vi "term_project.vi"() -> ()   [LabVIEW 2019]
uses:
  <vilib>/userdefined/High Color/IMAQdx.ctl
  <vilib>/Utility/file.llb/Read Delimited Spreadsheet (DBL).vi
  <vilib>/vision/driver/NI_Vision_Acquisition_Software.lvlib
  <vilib>/vision/NI_Vision_Development_Module.lvlib
panel:
  in  "Choose an Action":u16(ring) items=["RGB to Gray Conversion", "Gray to RGB Conversion", "Video Processing"]
  in  "Term Project Group 2":T1(tab)
  out "Time Passed (ms)":u32
  in  "Image Path RGBG":path=path "resources/lenacolored.png"
  out "Processed Gray Scale Image":T2(plugin-control)
  out "RGB Image":T2(plugin-control)
  out "Time Passed Labview (ms)":u32
  out "Labview Gray Scale Image":T2(plugin-control)
  in  "Colormap Circular Shift":i16(slide) scale=0.0..255.0
  out "Gray Scale Image":T2(plugin-control)
  out "Colored Image":T2(plugin-control)
  in  "Colormap File Path GRGB":path=path "resources/jet.csv"
  in  "Image Path GRGB":path=path "resources/lena.png"
  out "Time Passed":u32
  in  "Colormap Shift":i16(slide) scale=0.0..255.0
  in  "stop":bool
  in  "Choose Camera":T3="cam0"
  in  "Colormap File Path For Video":path=path "resources/parula.csv"
  out "Reproduced Image with Colormap":T2(plugin-control)
  out "Processed Image":T2(plugin-control)
  out "Captured Image":T2(plugin-control)
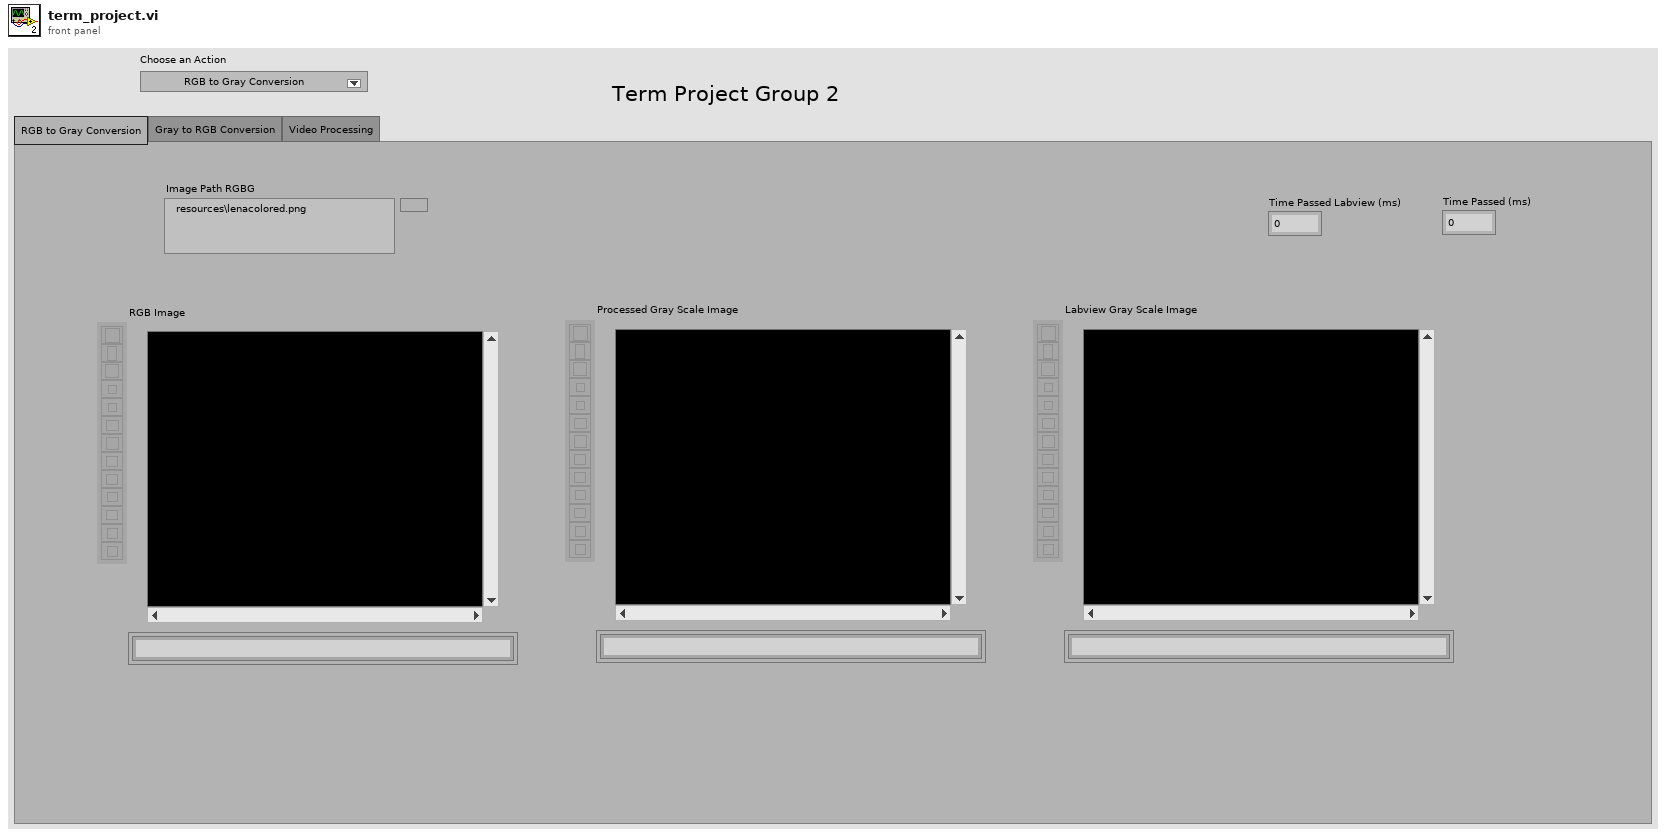
[diagram p1: front panel]
types:
  T1 = enum32{"RGB to Gray Conversion", "Gray to RGB Conversion", "Video Processing"}
  T2 = typedef "IMAQ Image.ctl" = refnum<image>
  T3 = typedef "IMAQdx.ctl" = refnum<k21>
  T4 = typedef "Image Type" = u32
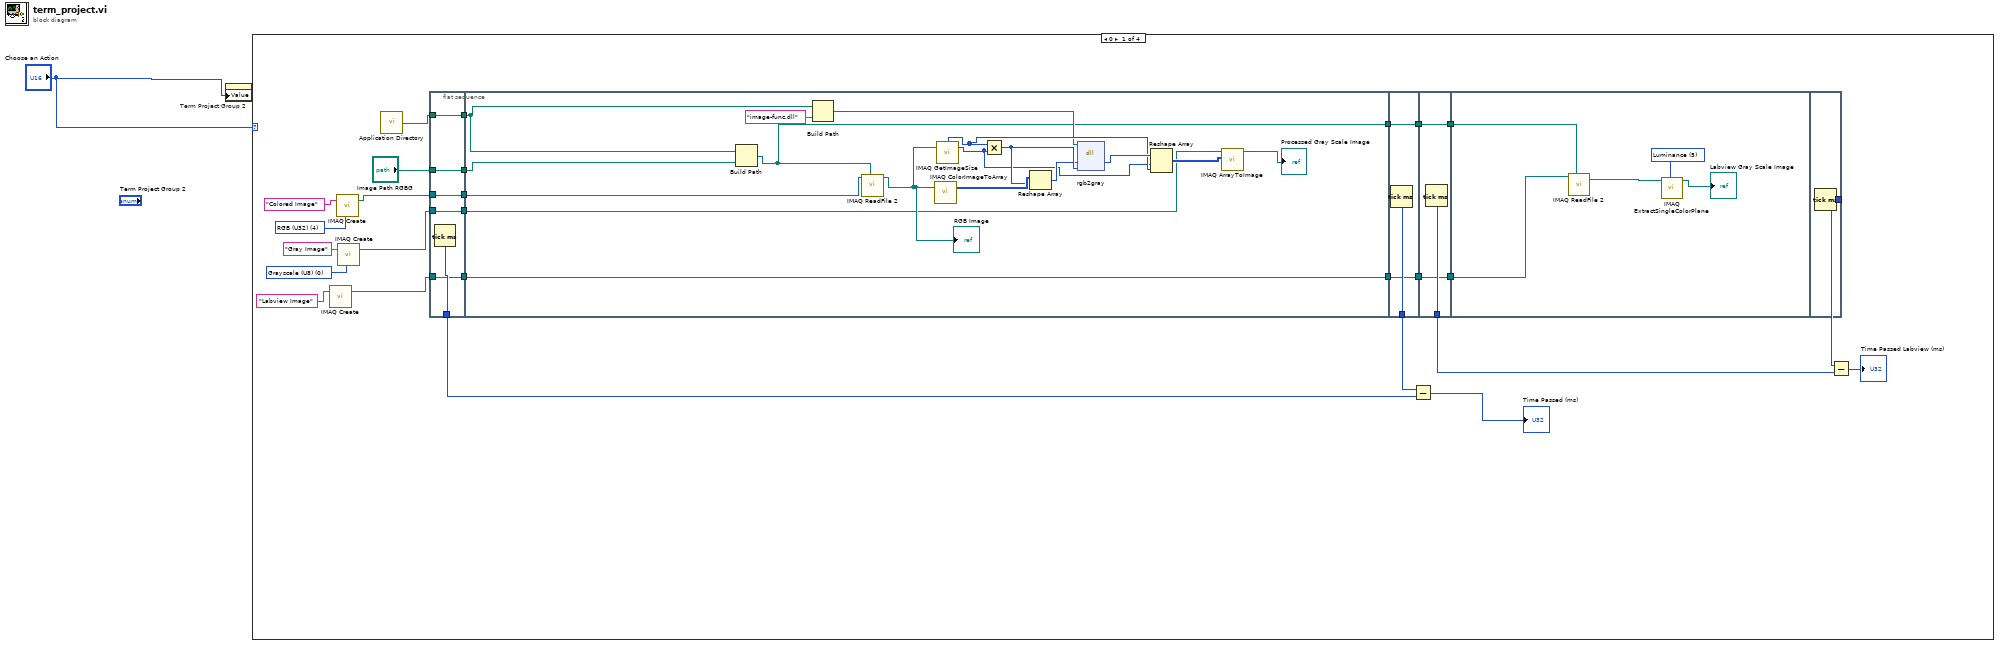
[diagram p0: block diagram]
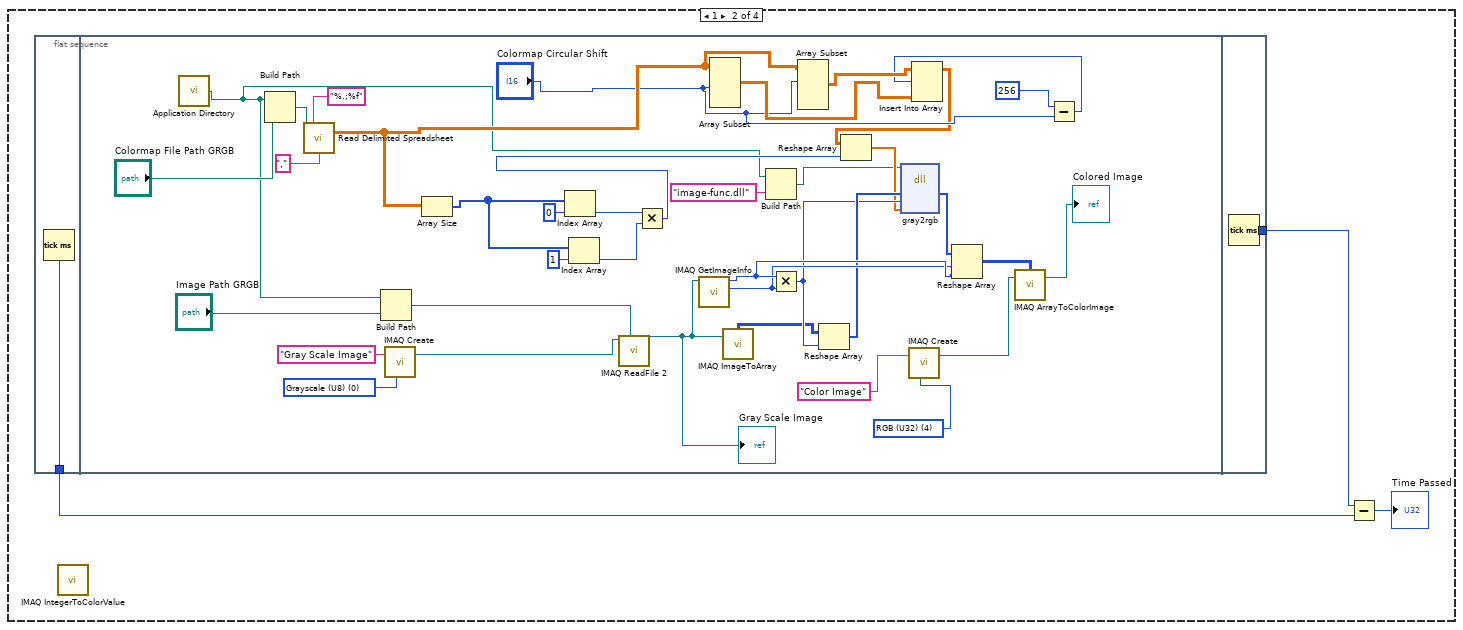
[diagram p2: hidden frame]
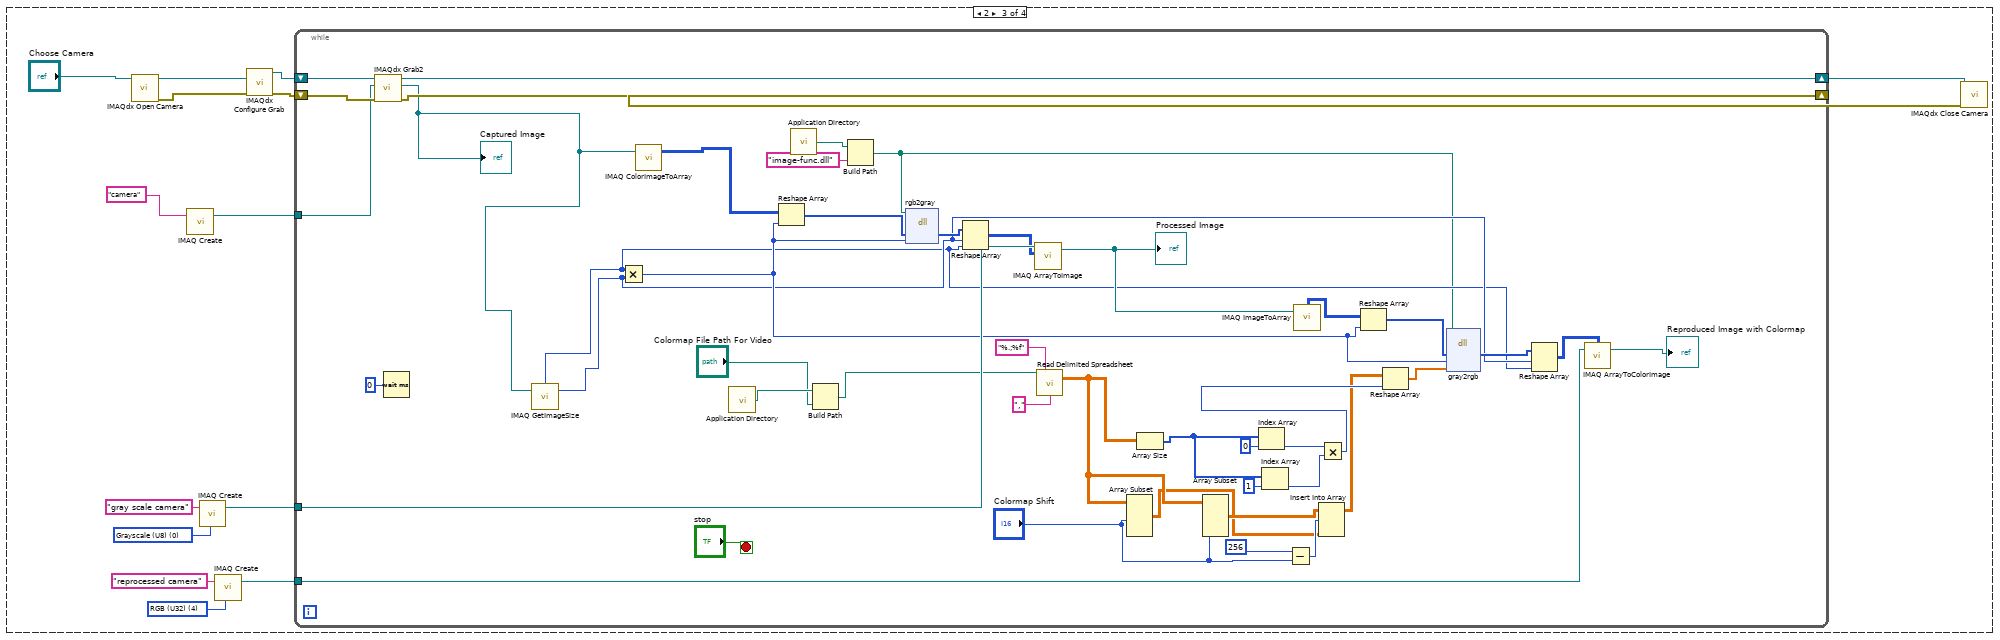
[diagram p3: hidden frame]
diagram:
  n1 = property on="Term Project Group 2" class="TabCtl (strict)"("Value"="Choose an Action") -> ()  [unwired: 2 in, 2 out]
  n2 = case shown="0" "Choose an Action" {
    frame 0 {
      w10 = T4 0 items=["Grayscale (U8)", "Grayscale (I16)", "Grayscale (SGL)", "Complex (CSG)", "RGB (U32)", "HSL (U32)", "RGB (U64)", "Grayscale (U16)"] ("Image Type")
      w14 = T4 4 items=["Grayscale (U8)", "Grayscale (I16)", "Grayscale (SGL)", "Complex (CSG)", "RGB (U32)", "HSL (U32)", "RGB (U64)", "Grayscale (U16)"] ("Image Type")
      n3 = call "IMAQ Create"("Image Name"="Labview Image") -> ("New Image"=w6:T2)  [unwired: 4 in, 1 out]
      n4 = call "IMAQ Create"("Image Name"="Colored Image", "Image Type"=w14) -> ("New Image"=w12:T2)  [unwired: 3 in, 1 out]
      n5 = call "IMAQ Create"("Image Name"="Gray Image", "Image Type"=w10) -> ("New Image"=w9:T2)  [unwired: 3 in, 1 out]
      n6 = call <vilib>:"Application Directory.vi"() -> ("Application Directory"=w18:path)
      n7 = flat-sequence {
        tunnel: [w34] -> w28
        tunnel: [w33] -> w19
        tunnel: w18 -> [w33]
        tunnel: [w32] -> w17
        tunnel: "Image Path RGBG" -> [w32]
        tunnel: [w31] -> w13
        tunnel: w12 -> [w31]
        tunnel: w9 -> [w30]
        tunnel: [w30] -> w8
        tunnel: w6 -> [w29]
        tunnel: [w29] -> w2
        tunnel: [w41] -> w25
        tunnel: w19 -> [w35]
        tunnel: w17 -> [w40]
        tunnel: w13 -> [w39]
        tunnel: w8 -> [w38]
        tunnel: [w37] -> w3
        tunnel: w2 -> [w37]
        tunnel: [w54] -> w26
        tunnel: w25 -> [w53]
        tunnel: [w53] -> w24
        tunnel: [w52] -> w4
        tunnel: w3 -> [w52]
        tunnel: w24 -> [w57]
        tunnel: [w57] -> w23
        tunnel: [w56] -> w22
        tunnel: [w55] -> w5
        tunnel: w4 -> [w55]
        tunnel: w23 -> [w62]
        tunnel: w5 -> [w61]
        tunnel: [w63] -> w21
        frame #0 {
          n8 = Tick Count (ms)() -> (millisecond timer value=w34:u32)
        }
        frame #1 {
          n9 = Build Path(base path=w35, name or relative path=w40) -> (appended path=w41:path)
          n10 = Build Path(base path=w35, name or relative path="image-func.dll") -> (appended path=w42:path)
          n11 = call "IMAQ ReadFile 2"("File Path"=w41, "Image"=w39) -> ("Image Out"=w44:T2)  [unwired: 5 in, 4 out]
          "RGB Image" <- w44
          n12 = call "IMAQ ColorImageToArray"("Image"=w44) -> ("Image Pixels (U32)"=w51:u32[][])  [unwired: 3 in, 2 out]
          n13 = call "IMAQ GetImageSize"("Image"=w44) -> ("Y Resolution"=w46:i32, "X Resolution"=w47:i32)  [unwired: 3 in, 1 out]
          n14 = Multiply(x=w47, y=w46) -> (x*y=w50:i32)
          n15 = Reshape Array(w51, w50) -> (w49:u32[])
          n16 = dll-call lib="C:/Users/User/Desktop/ee433 eben/image-func.dll" fn="rgb2gray"(path in=w42, "src"=w49, "total"=w50) -> ("src"=w48:i32[])  [unwired: 4 in, 2 out]
          n17 = Reshape Array(w48, w46, w47) -> (w45:i32[][])
          n18 = call "IMAQ ArrayToImage"("Image Pixels (U8)"=w45, "Image"=w38) -> ("Image Out"=→"Processed Gray Scale Image":T2)  [unwired: 8 in, 1 out]
        }
        frame #2 {
          n19 = Tick Count (ms)() -> (millisecond timer value=w54:u32)
        }
        frame #3 {
          n20 = Tick Count (ms)() -> (millisecond timer value=w56:u32)
        }
        frame #4 {
          w60 = 5 items=["Red", "Green", "Blue", "Hue", "Saturation", "Luminance", "Value", "Intensity"] ("Color Plane")
          n21 = call "IMAQ ReadFile 2"("File Path"=w62, "Image"=w61) -> ("Image Out"=w58:T2)  [unwired: 5 in, 4 out]
          n22 = call "IMAQ ExtractSingleColorPlane"("Color Plane"=w60, "Image Src"=w58) -> ("Image Dst Out"=→"Labview Gray Scale Image":T2)  [unwired: 8 in, 1 out]
        }
        frame #5 {
          n23 = Tick Count (ms)() -> (millisecond timer value=w63:u32)
        }
      }
      n24 = Subtract(x=w26, y=w28) -> (x-y=→"Time Passed (ms)":u32)
      n25 = Subtract(x=w21, y=w22) -> (x-y=→"Time Passed Labview (ms)":u32)
    }
    frame 1 {
      n26 = flat-sequence {
        tunnel: [w67] -> w65
        tunnel: [w106] -> w66
        frame #0 {
          n27 = Tick Count (ms)() -> (millisecond timer value=w67:u32)
        }
        frame #1 {
          w88 = T4 4 items=["Grayscale (U8)", "Grayscale (I16)", "Grayscale (SGL)", "Complex (CSG)", "RGB (U32)", "HSL (U32)", "RGB (U64)", "Grayscale (U16)"] ("Image Type")
          w86 = T4 0 items=["Grayscale (U8)", "Grayscale (I16)", "Grayscale (SGL)", "Complex (CSG)", "RGB (U32)", "HSL (U32)", "RGB (U64)", "Grayscale (U16)"] ("Image Type")
          n28 = call <vilib>:"Application Directory.vi"() -> ("Application Directory"=w71:path)
          n29 = Build Path(base path=w71, name or relative path="Colormap File Path GRGB") -> (appended path=w75:path)
          n30 = call-poly <vilib>:"Read Delimited Spreadsheet.vi"("file path (dialog if empty)"=w75, "format (%.3f)"="%.;%f", "delimiter (\\t)"="," ("delimiter (\\t)")) -> ("all rows"=w82:dbl[][])  [unwired: 7 in, 5 out]
          n31 = Build Path(base path=w71, name or relative path="Image Path GRGB") -> (appended path=w70:path)
          n32 = call "IMAQ Create"("Image Name"="Gray Scale Image", "Image Type"=w86) -> ("New Image"=w94:T2)  [unwired: 3 in, 1 out]
          n33 = Array Size(array=w82) -> (size(s)=w90:i32[])
          n34 = Index Array(array=w90, index=0) -> (element=w91:i32)
          n35 = Index Array(array=w90, index=1) -> (element=w92:i32)
          n36 = call "IMAQ ReadFile 2"("File Path"=w70, "Image"=w94) -> ("Image Out"=w105:T2)  [unwired: 5 in, 4 out]
          "Gray Scale Image" <- w105
          n37 = Multiply(x=w91, y=w92) -> (x*y=w93:i32)
          n38 = call "IMAQ GetImageInfo"("Image"=w105) -> ("Y Resolution"=w101:i32, "X Resolution"=w102:i32)  [unwired: 3 in, 6 out]
          n39 = Array Subset(array=w82, length (row)="Colormap Circular Shift") -> (w80:dbl[][])  [unwired: 3 in]
          n40 = call "IMAQ ImageToArray"("Image"=w105) -> ("Image Pixels (U8)"=w96:u8[][])  [unwired: 3 in, 4 out]
          n41 = Build Path(base path=w71, name or relative path="image-func.dll") -> (appended path=w73:path)
          n42 = Multiply(x=w102, y=w101) -> (x*y=w97:i32)
          n43 = Array Subset(array=w82, index (row)="Colormap Circular Shift") -> (w81:dbl[][])  [unwired: 3 in]
          n44 = Reshape Array(w96, w97) -> (w98:u8[])
          n45 = call "IMAQ Create"("Image Name"="Color Image", "Image Type"=w88) -> ("New Image"=w104:T2)  [unwired: 3 in, 1 out]
          n46 = Subtract(x=256, y="Colormap Circular Shift") -> (x-y=w78:i32)
          n47 = Insert Into Array(array=w81, index (row)=w78, new element=w80) -> (w69:dbl[][])  [unwired: 1 in]
          n48 = Reshape Array(w69, w93) -> (w95:dbl[])
          n49 = dll-call lib="C:/Users/User/Desktop/ee433 eben/image-func.dll" fn="gray2rgb"(path in=w73, "src"=w98, "total"=w97, "colormap"=w95) -> ("src"=w103:i32[])  [unwired: 5 in, 2 out]
          n50 = Reshape Array(w103, w101, w102) -> (w100:i32[][])
          n51 = call "IMAQ ArrayToColorImage"("Image Pixels (U32)"=w100, "Image"=w104) -> ("Image Out"=→"Colored Image":T2)  [unwired: 3 in, 1 out]
        }
        frame #2 {
          n52 = Tick Count (ms)() -> (millisecond timer value=w106:u32)
        }
      }
      n53 = call "IMAQ IntegerToColorValue"() -> ()  [unwired: 5 in, 4 out]
      n54 = Subtract(x=w66, y=w65) -> (x-y=→"Time Passed":u32)
    }
    frame 2 {
      w108 = T4 4 items=["Grayscale (U8)", "Grayscale (I16)", "Grayscale (SGL)", "Complex (CSG)", "RGB (U32)", "HSL (U32)", "RGB (U64)", "Grayscale (U16)"] ("Image Type")
      w111 = T4 0 items=["Grayscale (U8)", "Grayscale (I16)", "Grayscale (SGL)", "Complex (CSG)", "RGB (U32)", "HSL (U32)", "RGB (U64)", "Grayscale (U16)"] ("Image Type")
      n55 = call <vilib>:"IMAQdx Open Camera.vi"("Session In"="Choose Camera") -> ("error out"=w117:errorcluster, "Session Out"=w121:T3)  [unwired: 9 in]
      n56 = call "IMAQ Create"("Image Name"="camera") -> ("New Image"=w113:T2)  [unwired: 4 in, 1 out]
      n57 = call "IMAQ Create"("Image Name"="gray scale camera", "Image Type"=w111) -> ("New Image"=w110:T2)  [unwired: 3 in, 1 out]
      n58 = call "IMAQ Create"("Image Name"="reprocessed camera", "Image Type"=w108) -> ("New Image"=w107:T2)  [unwired: 3 in, 1 out]
      n59 = call <vilib>:"IMAQdx Configure Grab.vi"("error in"=w117, "Session In"=w121) -> ("error out"=w116:errorcluster, "Session Out"=w120:T3)  [unwired: 8 in]
      n60 = while {
        tunnel: w113 -> [w160]
        shift-right: [w165] -> w119
        shift-left: w120 -> [w166]
        shift-right: [w163] -> w115
        shift-left: w116 -> [w164]
        tunnel: w110 -> [w157]
        tunnel: w107 -> [w138]
        stop <- "stop" stop-if-true
        n61 = call <vilib>:"IMAQdx Grab2.vi"("error in"=w164, "Image In"=w160, "Session In"=w166) -> ("error out"=w163:errorcluster, "Image Out"=w159:T2, "Session Out"=w165:T3)  [unwired: 5 in, 1 out]
        "Captured Image" <- w159
        n62 = Wait (ms)(milliseconds to wait=u32 0) -> ()  [unwired: 1 out]
        n63 = call "IMAQ GetImageSize"("Image"=w159) -> ("Y Resolution"=w140:i32, "X Resolution"=w139:i32)  [unwired: 3 in, 1 out]
        n64 = Multiply(x=w139, y=w140) -> (x*y=w142:i32)
        n65 = call "IMAQ ColorImageToArray"("Image"=w159) -> ("Image Pixels (U32)"=w158:u32[][])  [unwired: 3 in, 2 out]
        n66 = call <vilib>:"Application Directory.vi"() -> ("Application Directory"=w125:path)
        n67 = Reshape Array(w158, w142) -> (w155:u32[])
        n68 = call <vilib>:"Application Directory.vi"() -> ("Application Directory"=w128:path)
        n69 = Build Path(base path=w125, name or relative path="Colormap File Path For Video") -> (appended path=w123:path)
        n70 = Build Path(base path=w128, name or relative path="image-func.dll") -> (appended path=w126:path)
        n71 = dll-call lib="C:/Users/User/Desktop/ee433 eben/image-func.dll" fn="rgb2gray"(path in=w126, "src"=w155, "total"=w142) -> ("src"=w154:i32[])  [unwired: 4 in, 2 out]
        n72 = Reshape Array(w154, w140, w139) -> (w156:i32[][])
        n73 = call "IMAQ ArrayToImage"("Image Pixels (U8)"=w156, "Image"=w157) -> ("Image Out"=w145:T2)  [unwired: 8 in, 1 out]
        "Processed Image" <- w145
        n74 = call-poly <vilib>:"Read Delimited Spreadsheet.vi"("file path (dialog if empty)"=w123, "format (%.3f)"="%.;%f", "delimiter (\\t)"="," ("delimiter (\\t)")) -> ("all rows"=w135:dbl[][])  [unwired: 7 in, 5 out]
        n75 = Array Subset(array=w135, length (row)="Colormap Shift") -> (w130:dbl[][])  [unwired: 3 in]
        n76 = Array Size(array=w135) -> (size(s)=w151:i32[])
        n77 = Array Subset(array=w135, index (row)="Colormap Shift") -> (w131:dbl[][])  [unwired: 3 in]
        n78 = Index Array(array=w151, index=0) -> (element=w149:i32)
        n79 = Index Array(array=w151, index=1) -> (element=w148:i32)
        n80 = Subtract(x=i16 256, y="Colormap Shift") -> (x-y=w132:i16)
        n81 = call "IMAQ ImageToArray"("Image"=w145) -> ("Image Pixels (U8)"=w144:u8[][])  [unwired: 3 in, 4 out]
        n82 = Insert Into Array(array=w131, index (row)=w132, new element=w130) -> (w129:dbl[][])  [unwired: 1 in]
        n83 = Multiply(x=w149, y=w148) -> (x*y=w147:i32)
        n84 = Reshape Array(w144, w142) -> (w143:u8[])
        n85 = Reshape Array(w129, w147) -> (w146:dbl[])
        n86 = dll-call lib="C:/Users/User/Desktop/ee433 eben/image-func.dll" fn="gray2rgb"(path in=w126, "src"=w143, "total"=w142, "colormap"=w146) -> ("src"=w141:i32[])  [unwired: 5 in, 2 out]
        n87 = Reshape Array(w141, w140, w139) -> (w137:i32[][])
        n88 = call "IMAQ ArrayToColorImage"("Image Pixels (U32)"=w137, "Image"=w138) -> ("Image Out"=→"Reproduced Image with Colormap":T2)  [unwired: 3 in, 1 out]
      }
      n89 = call <vilib>:"IMAQdx Close Camera.vi"("error in"=w115, "Session In"=w119) -> ()  [unwired: 9 in, 1 out]
    }
    frame Default {
    }
  }
